vi "Get Document Reference.vi"(8 "error in (no error)":errorcluster, 11 "ooWriter in":refnum<class "ooWriter.lvclass">) -> (0 "error out":errorcluster, 1 "Document":refnum<k24>, 3 "ooWriter out":refnum<class "ooWriter.lvclass">)   [LabVIEW 2009, in "ooWriter.lvclass"]
uses:
  ooWriter.lvclass
  C:/Projets/LAVAG/OpenOfficeRGT/AODL/DLLs/AODL.dll
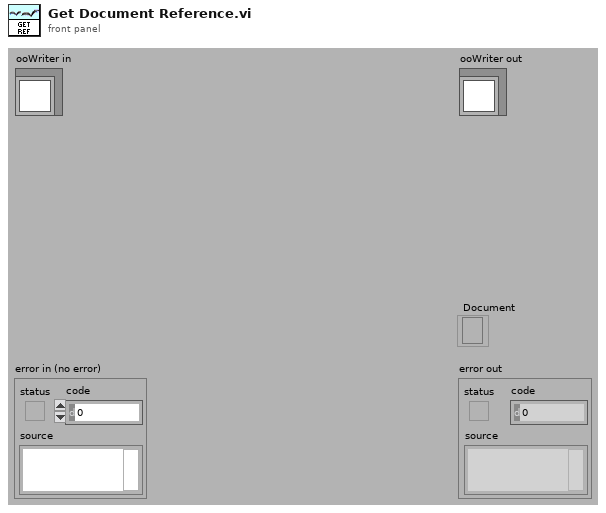
[diagram p1: front panel]
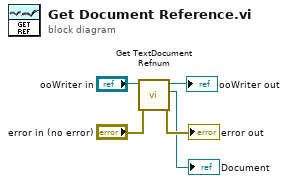
[diagram p0: block diagram]
diagram:
  n1 = call-dynamic "Get TextDocument Refnum.vi"("error in (no error)"="error in (no error)", "ooWriter in"="ooWriter in") -> ("error out"=→"error out":errorcluster, "TextDocument"=→"Document":refnum<k24>, "ooWriter out"=→"ooWriter out":refnum<class "ooWriter.lvclass">)  [unwired: 7 in]
